vi "SP Convert Frequency from MHz Array.vi"(10 "Units":T1=enum."MHz", 11 "Frequency Array":dbl[](array[numeric])) -> (3 "Converted Frequency Array":dbl[](array[numeric]))   [LabVIEW 2011]
uses:
  TypeDefs/SP Frequency Units.ctl
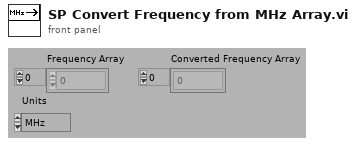
[diagram p1: front panel]
types:
  T1 = typedef "SP Frequency Units.ctl" = enum16{"Hz", "kHz", "MHz", "GHz", "Points"}
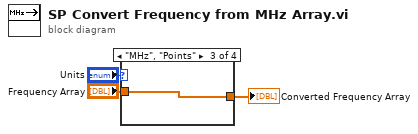
[diagram p0: block diagram]
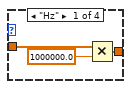
[diagram p2: hidden frame]
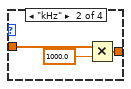
[diagram p3: hidden frame]
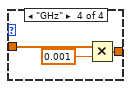
[diagram p4: hidden frame]
diagram:
  n1 = case shown="\"MHz\", \"Points\"" "Units" {
    tunnel: "Frequency Array" -> [w6 w9 w10 w13]
    tunnel: [w5 w8 w10 w12] -> w3
    frame "Hz" {
      n2 = Multiply(x=w6, y=1000000.0) -> (x*y=w5:dbl[])
    }
    frame "kHz" {
      n3 = Multiply(x=w9, y=1000.0) -> (x*y=w8:dbl[])
    }
    frame "MHz", "Points" {
    }
    frame "GHz" {
      n4 = Multiply(x=w13, y=0.001) -> (x*y=w12:dbl[])
    }
  }
  "Converted Frequency Array" <- w3
